vi "Open Close Device.vi"(11 "Device Name":string="Basys2") -> (0 "Error Out":errorcluster, 3 "HIF":u32)   [LabVIEW 2011, in "LVH-Adept.lvlib"]
uses:
  LVH-Adept.lvlib
  Private/DMGR/DMGR.lvlib
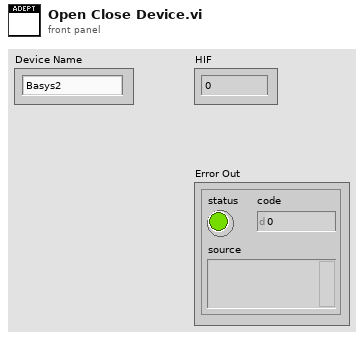
[diagram p1: front panel]
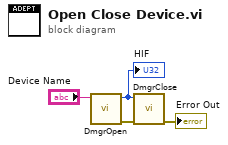
[diagram p0: block diagram]
diagram:
  n1 = call "DmgrOpen.vi"("Device Name"="Device Name") -> ("Error Out"=w4:errorcluster, "Device Handle"=w3:u32)  [unwired: 9 in]
  "HIF" <- w3
  n2 = call "DmgrClose.vi"("Error In"=w4, "hif"=w3) -> ("Error Out"=→"Error Out":errorcluster)  [unwired: 9 in]
